vi "SCPI Cmd.vi"(0 "VISA资源名称":refnum<visa-resource-name>, 1 "缓存区大小":u32, 2 "SCPI字符串":string, 3 "错误输入（无错误）":errorcluster) -> (7 "VISA资源名称输出":refnum<visa-resource-name>, 8 "读取缓冲区":string, 9 "返回数":u32, 10 "错误输出":errorcluster)   [LabVIEW 2018]
doc: "SCPI操作命令"
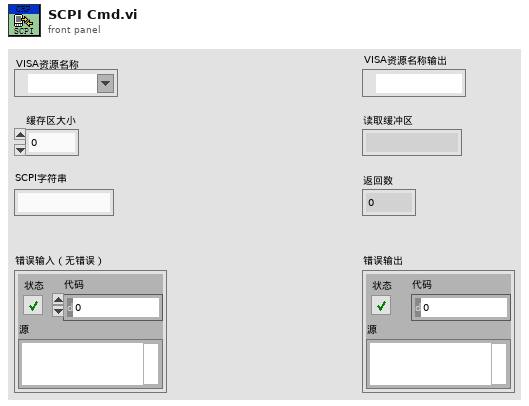
[diagram p1: front panel]
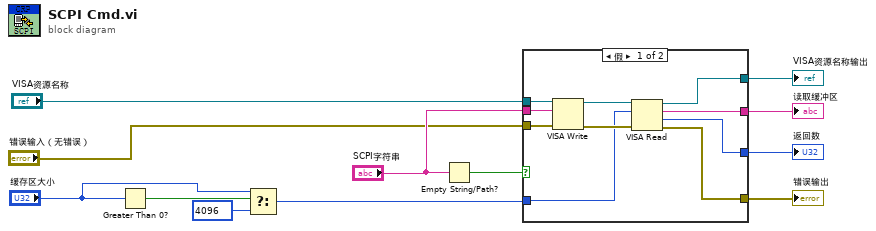
[diagram p0: block diagram]
diagram:
  n1 = Greater Than 0?(x="缓存区大小") -> (x > 0?=w12:bool)
  n2 = Select(t="缓存区大小", s=w12, f=u32 4096) -> (s? t:f=w5:u32)
  n3 = Empty String/Path?(string/path="SCPI字符串") -> (empty?=w9:bool)
  n4 = case shown="假" w9 {
    tunnel: "VISA资源名称" -> [w22 w24]
    tunnel: "SCPI字符串" -> [w21 _]
    tunnel: "错误输入（无错误）" -> [w20 w23]
    tunnel: [w17 w23] -> w7
    tunnel: [w16 w24] -> w6
    tunnel: w5 -> [w15 _]
    tunnel: [w14 _] -> w4
    tunnel: [w13 _] -> w3
    frame False {
      n5 = VISA Write(VISA resource name=w22, write buffer=w21, error in (no error)=w20) -> (VISA resource name out=w19:refnum<visa-resource-name>, error out=w18:errorcluster)  [unwired: 1 out]
      n6 = VISA Read(VISA resource name=w19, byte count=w15, error in (no error)=w18) -> (VISA resource name out=w16:refnum<visa-resource-name>, read buffer=w14:string, return count=w13:u32, error out=w17:errorcluster)
    }
    frame True {
    }
  }
  "错误输出" <- w7
  "VISA资源名称输出" <- w6
  "读取缓冲区" <- w4
  "返回数" <- w3
